vi "Size Constants.vi"() -> (2 "Size Constants":T1)   [LabVIEW 2022 SP3, in "FlexBlocks Support.lvlib"]
uses:
  FlexBlocks Support.lvlib
  Size Constants.ctl
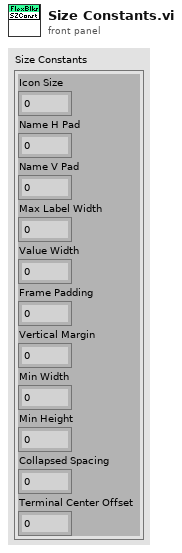
[diagram p1: front panel]
types:
  T1 = typedef "FlexBlocks Support.lvlib/Size Constants.ctl" = cluster{"Icon Size":i32, "Name H Pad":i32, "Name V Pad":i32, "Max Label Width":i32, "Value Width":i32, "Frame Padding":i32, "Vertical Margin":i32, "Min Width":i32, "Min Height":i32, "Collapsed Spacing":i32, "Terminal Center Offset":i32}
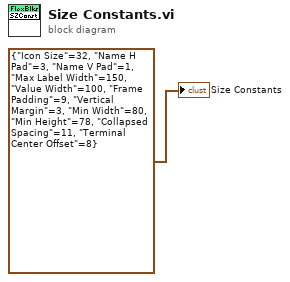
[diagram p0: block diagram]
diagram:
  "Size Constants" <- T1 {"Icon Size"=32, "Name H Pad"=3, "Name V Pad"=1, "Max Label Width"=150, "Value Width"=100, "Frame Padding"=9, "Vertical Margin"=3, "Min Width"=80, "Min Height"=78, "Collapsed Spacing"=11, "Terminal Center Offset"=8} ("Size Constants")
